vi "Read Port.vi"(8 "error in":errorcluster, 11 "TCP slave in":refnum<class "TCP Server.lvclass">) -> (0 "error out":errorcluster, 2 "Port":u16, 3 "TCP slave out":refnum<class "TCP Server.lvclass">)   [LabVIEW 2021, in "WebSockets.lvlib" / "TCP Server.lvclass"]
doc: "Property accessor for the TCP port."
uses:
  TCP Server.lvclass
  D:/my_projects/projects/Algorithms/Labview/21/WebSockets/WebSockets/WebSocket/WebSocket.lvclass
  WebSocket/WebSocket.lvclass/WebSocket.ctl
  Sockets/VISA TCP Socket/VISA TCP.lvclass
  Sockets/VISA TCP Socket/VISA TCP.lvclass/VISA TCP.ctl
  Sockets/Socket/Socket.lvclass
  WebSocket/WebSocket.lvclass
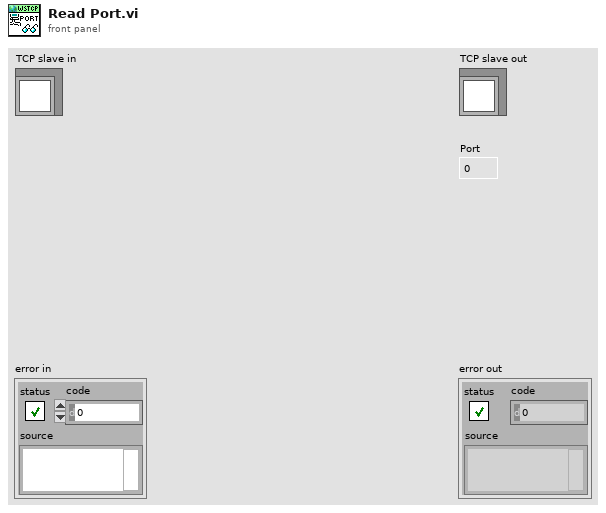
[diagram p1: front panel]
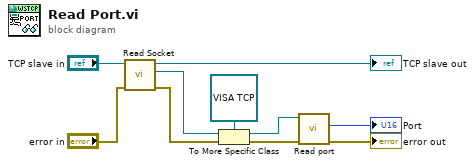
[diagram p0: block diagram]
diagram:
  n1 = call "Read Socket.vi"("error in (no error)"="error in", "WebSocket in"="TCP slave in") -> ("error out"=w3:errorcluster, "Socket"=w9:refnum<class "Socket.lvclass">, "WebSocket out"=→"TCP slave out":refnum<class "TCP Server.lvclass">)  [unwired: 7 in]
  n2 = To More Specific Class(target class=refnum<class "VISA TCP.lvclass"> refnum ("Sockets:VISA TCP"), reference=w9, error in=w3) -> (specific class reference=w8:refnum<class "VISA TCP.lvclass">, error out=w2:errorcluster)
  n3 = call "Read port.vi"("error in (no error)"=w2, "VISA TCP in"=w8) -> ("error out"=→"error out":errorcluster, "port"=→"Port":u16)  [unwired: 7 in, 1 out]
